vi "lookupService.vi"(6 "Parameters":T2={"Caller ID"="/labview", "Topic"="/topic", "Topic Type"="topic type", "Caller API"="API"}) -> (0 "Reply":T1, 2 "lookupService":string="POST /RPC2 HTTP/1.1\r\nHost: 192.168.1.110:11311\r\nContent-Type: text/xml\r\nContent-Length: 396\r\n\r\n<?xml version='1.0'?>\n<methodCall>\r <methodName>registerSubscriber</methodName>\r <params>\r   <param><value><string>/ChrisAir</string> </value> </param>\r   <param><value><string>/robot/joint_states</string> </value> </param>\r   <param><value><string>sensor_msgs/JointState</string> </value> </param>\r   <param><value><string>http://192.168.1.111</string> </value> </param>\r </params>\r</methodCall>", 3 "response":string, 5 "error out":errorcluster)   [LabVIEW 2013]
uses:
  _ROSDefinition.vi
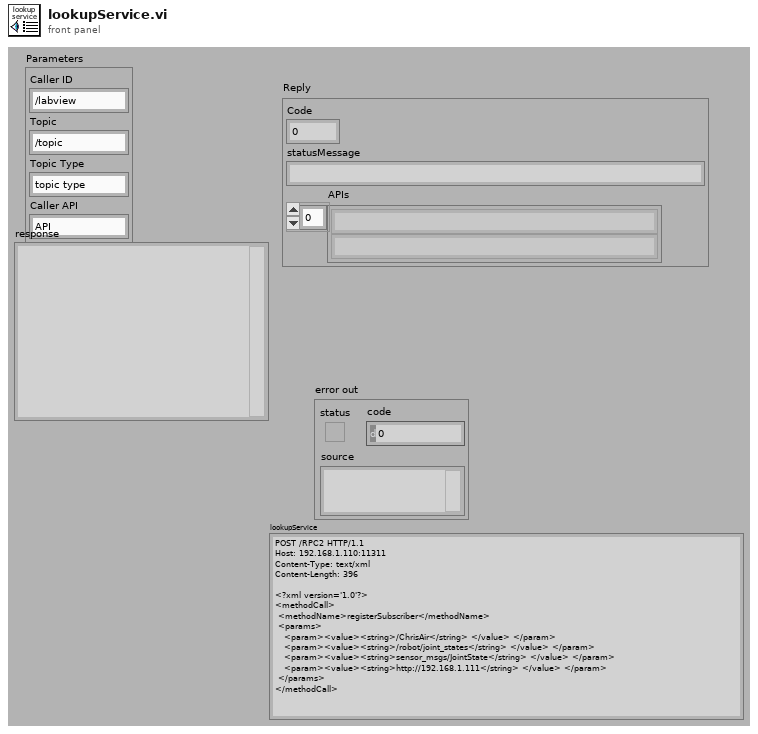
[diagram p1: front panel]
types:
  T1 = cluster{"Code":i8, "statusMessage":string, "APIs":string[]}
  T2 = cluster{"Caller ID":string, "Topic":string, "Topic Type":string, "Caller API":string}
  T3 = cluster{"Code":i8, "statusMessage":string, "APIs":string[]}[]
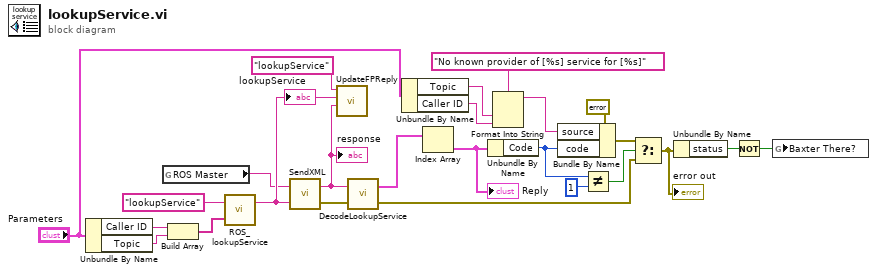
[diagram p0: block diagram]
diagram:
  n1 = Unbundle By Name("Parameters") -> ("Caller ID"=w25:string, "Topic"=w24:string)
  n2 = global read "_ROSDefinition.vi" "ROS Master"() -> (w1:string)
  n3 = Build Array(w25, w24) -> (w23:string[])
  n4 = call "ROS_lookupService.vi"("Parameters"=w23, "Method Name"="lookupService") -> ("lookupService"=w19:string)  [unwired: 1 in]
  "lookupService" <- w19
  n5 = call "SendXML.vi"("Send"=w19, "URI in"=w1) -> ("error out"=w21:errorcluster, "Reply"=w18:string)
  "response" <- w18
  n6 = call "UpdateFPReply.vi"("Reply"=w18, "Sent"=w19, "method"="lookupService" ("Method Name")) -> ()  [unwired: 3 in]
  n7 = call "DecodeLookupService.vi"("error in (no error)"=w21, "Response"=w18) -> ("error out"=w7:errorcluster, "Reply 2"=w20:T3)
  n8 = Unbundle By Name("Parameters") -> ("Topic"=w4:string, "Caller ID"=w3:string)
  n9 = Index Array(array=w20) -> (element=w9:T1)  [unwired: 1 in]
  "Reply" <- w9
  n10 = Unbundle By Name(w9) -> ("Code"=w11:i8)
  n11 = Format Into String(format string="No known provider of [%s] service for [%s]", w4, w3) -> (resulting string=w2:string)  [unwired: 2 in, 1 out]
  n12 = Bundle By Name(cluster=errorcluster {"status"=TRUE, "code"=0, "source"=" Error"} ("t"), "source"=w2, "code"=w11) -> (w10:errorcluster)
  n13 = Not Equal?(x=w11, y=i8 1) -> (x != y?=w13:bool)
  n14 = Select(t=w10, s=w13, f=w7) -> (s? t:f=w8:errorcluster)
  "error out" <- w8
  n15 = Unbundle By Name(w8) -> ("status"=w15:bool)
  n16 = Not(x=w15) -> (.not. x?=w16:bool)
  n17 = global write "_ROSDefinition.vi" "Baxter There?"(w16) -> ()
